vi "Untitled 1.vi"(8 "error in (no error)":errorcluster, 11 "4081 in":refnum<class "4081.lvclass">) -> (0 "error out":errorcluster, 3 "4081 out":refnum<class "4081.lvclass">)   [LabVIEW 2019, in "4081.lvlib" / "4081.lvclass"]
uses:
  4081.lvclass
  <instrlib>/niDMM/nidmm.llb/niDMM Configure Measurement Digits.vi
  <instrlib>/niDMM/nidmm.llb/niDMM Read Waveform (waveform data).vi
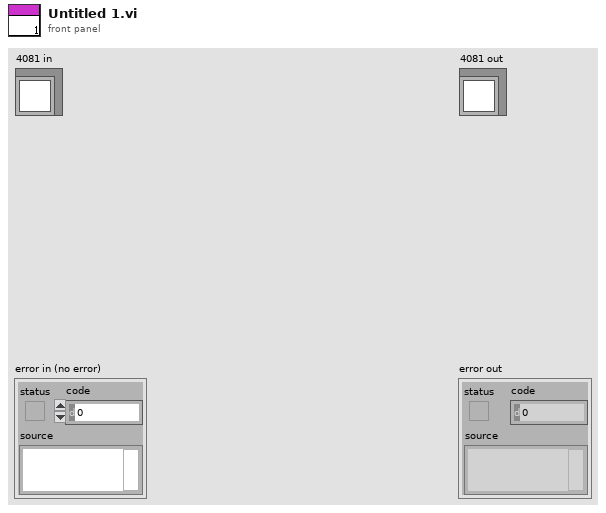
[diagram p1: front panel]
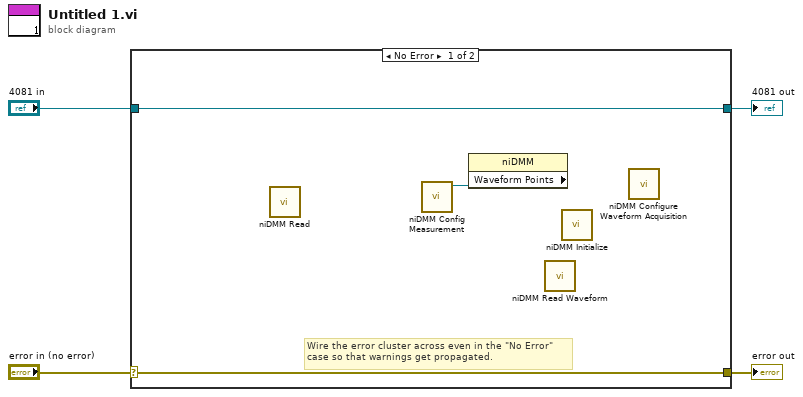
[diagram p0: block diagram]
diagram:
  n1 = case shown="No Error" "error in (no error)" {
    selector: "error in (no error)" -> [w6 w9]
    tunnel: [w6 w9] -> w3
    tunnel: [w7 w8] -> w1
    tunnel: "4081 in" -> [w7 w8]
    frame No Error {
      # "Wire the error cluster across even in the \"No Error\"\ncase so that warnings get propagated."
      n2 = call <instrlib>:"niDMM Read.vi"() -> ()  [unwired: 9 in, 3 out]
      n3 = call-poly <instrlib>:"niDMM Config Measurement.vi"() -> ("instrument handle out"=w5:refnum<k15>)  [unwired: 10 in, 1 out]
      n4 = property class="niDMM" props=["Waveform Points"](reference=w5) -> ()  [unwired: 1 in, 3 out]
      n5 = call-poly <instrlib>:"niDMM Read Waveform.vi"() -> ()  [unwired: 8 in, 4 out]
      n6 = call <instrlib>:"niDMM Initialize.vi"() -> ()  [unwired: 10 in, 2 out]
      n7 = call <instrlib>:"niDMM Configure Waveform Acquisition.vi"() -> ()  [unwired: 10 in, 2 out]
    }
    frame Error {
    }
  }
  "error out" <- w3
  "4081 out" <- w1
